vi "参数设置页.vi"() -> ()   [LabVIEW 2016, in "斯坦道CODMn.lvlib"]
panel:
  in  "手动模式":bool
  in  "采水泵排液时间/s:":i32
  in  "采水泵沉淀时间/s:":i32
  in  "采水泵润洗时间/s:":i32
  in  "采水泵进样时间/s:":i32
  in  "标度泵计量数 2":dbl
  in  "零点泵计量数 2":dbl
  in  "氢氧化钠:":dbl
  in  "屏蔽负值":bool
  in  "常规版/认证版":enum16{"常规版-酸性", "常规版-碱性", "认证版", "浮台版"}(ring)
  out "稀释倍数解释":string
  in  "CODMn零点核查选择":enum16{"零点核查走纯水管", "零点核查走零漂管"}(ring)
  in  "低量程稀释倍数:":dbl=1.0
  in  "高量程稀释倍数:":dbl=2.0
  in  "零点液自动补测":bool
  in  "跨度液自动补测":bool
  in  "标准液自动补测":bool
  in  "零点液偏差":dbl
  in  "跨度液偏差":dbl
  in  "标准液偏差":dbl
  in  "更换泵管":bool
  in  "跨度值":dbl
  in  "加标回收量程：":enum32{"H", "L", "AUTO"}(ring)=enum."AUTO"
  out "CODMn序列号":string
  out "CODMn软件版本：":string
  in  "标样核查量程选择":enum32{"H", "L", "AUTO"}(ring)=enum."AUTO"
  in  "标样浓度":dbl
  in  "零点核查量程选择":enum32{"H", "L", "AUTO"}(ring)=enum."AUTO"
  in  "零点核查浓度":dbl
  in  "跨度量程选择":enum32{"H", "L", "AUTO"}(ring)=enum."AUTO"
  in  "跨度液浓度":dbl
  in  "水样：":dbl
  in  "蒸馏水：":dbl
  in  "标液：":dbl
  in  "零点核查样：":dbl
  in  "加标回收样：":dbl
  in  "草酸钠":dbl
  in  "高锰酸钾":dbl
  in  "硫酸":dbl
  out "量程解释说明":string
  in  "高切低阈值:":dbl
  in  "低切高阈值:":dbl
  in  "水样量程选择:":enum16{"L", "H", "自动切换测一次", "自动切换测两次"}(ring)
  in  "标准液浓度":dbl
  in  "温度":dbl
  in  "恒温时间":dbl
  in  "当前量程：":enum16{"L", "H"}(ring)
  # "基本参数设置"
  # "泵计量参数设置"
  # "高锰酸钾："
  # "加热恒温温度(℃):"
  # "草酸钠："
  # "恒温时间(分钟):"
  # "硫酸："
  # "标准液浓度(mg/L):"
  # "跨度核查浓度："
  # "零点液偏差±:"
  # "标准液偏差%:"
  # "跨度核查量程："
  # "跨度液偏差%:"
  # "零点核查浓度："
  # "标样浓度："
  # "零点核查量程："
  # "标样核查量程："
  # "跨度值:"
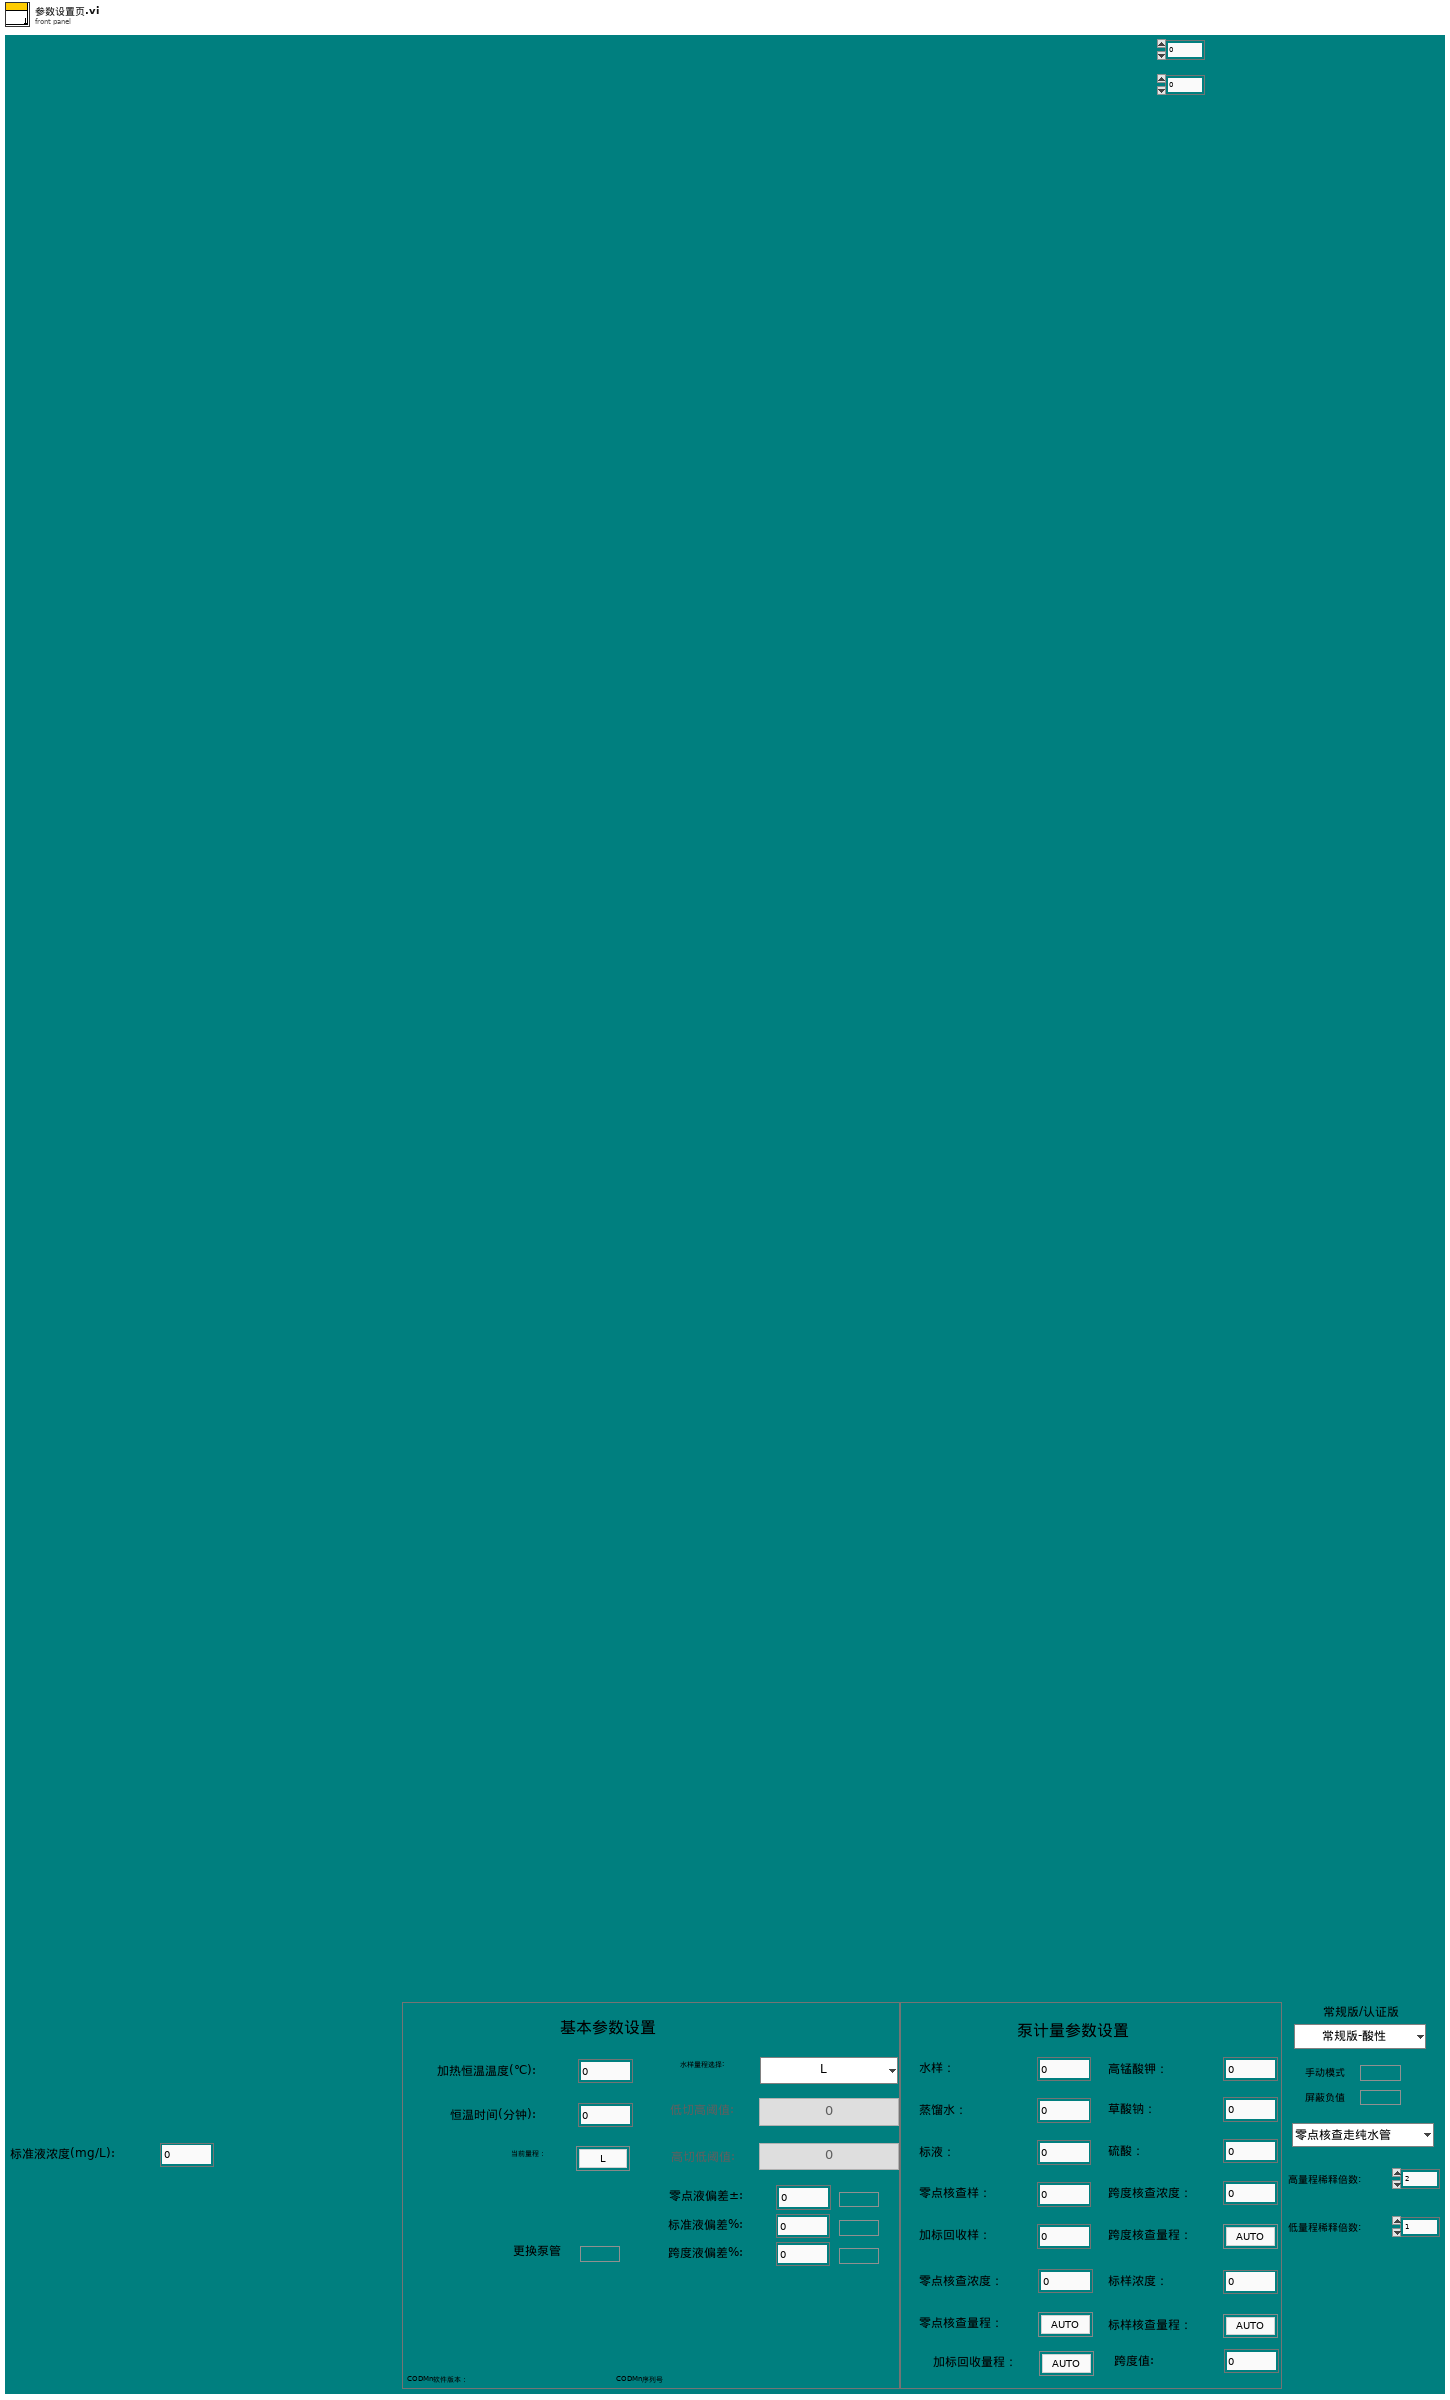
[diagram p1: front panel]
types:
  T1 = cluster{"时间":timestamp, "水样计量数":u16, "蒸馏水计量数":u16, "标液计量数":u16, "零点核查计量数":u16, "加标回收计量数":u16, "硫酸计量数":u16, "高锰酸钾计量数":u16, "草酸钠计量数":u16, "更换泵管":string}
  T2 = cluster{"测量量程":dbl, "测量精度":dbl, "测量间隔":dbl, "消解温度":dbl, "消解时长":dbl, "空白校准时间":timestamp, "曲线截距":dbl, "曲线斜率":dbl, "测量检出限":dbl, "测量信号值":dbl, "线性相关系数":dbl, "二次多项式系数":dbl, "标样校准时间":timestamp, "稀释倍数":dbl, "三项式系数":dbl, "空白标定系数":dbl, "量程系数":dbl, "F0/ORPA":dbl, "F1/ORPB":dbl, "F2/ORPK":dbl, "F3":dbl, "F4":dbl, "F5":dbl, "F6":dbl, "F7":dbl, "X0/滴定数":dbl, "量程":dbl}
  T3 = enum8{"Enabled", "Disabled", "Disabled and Grayed Out"}
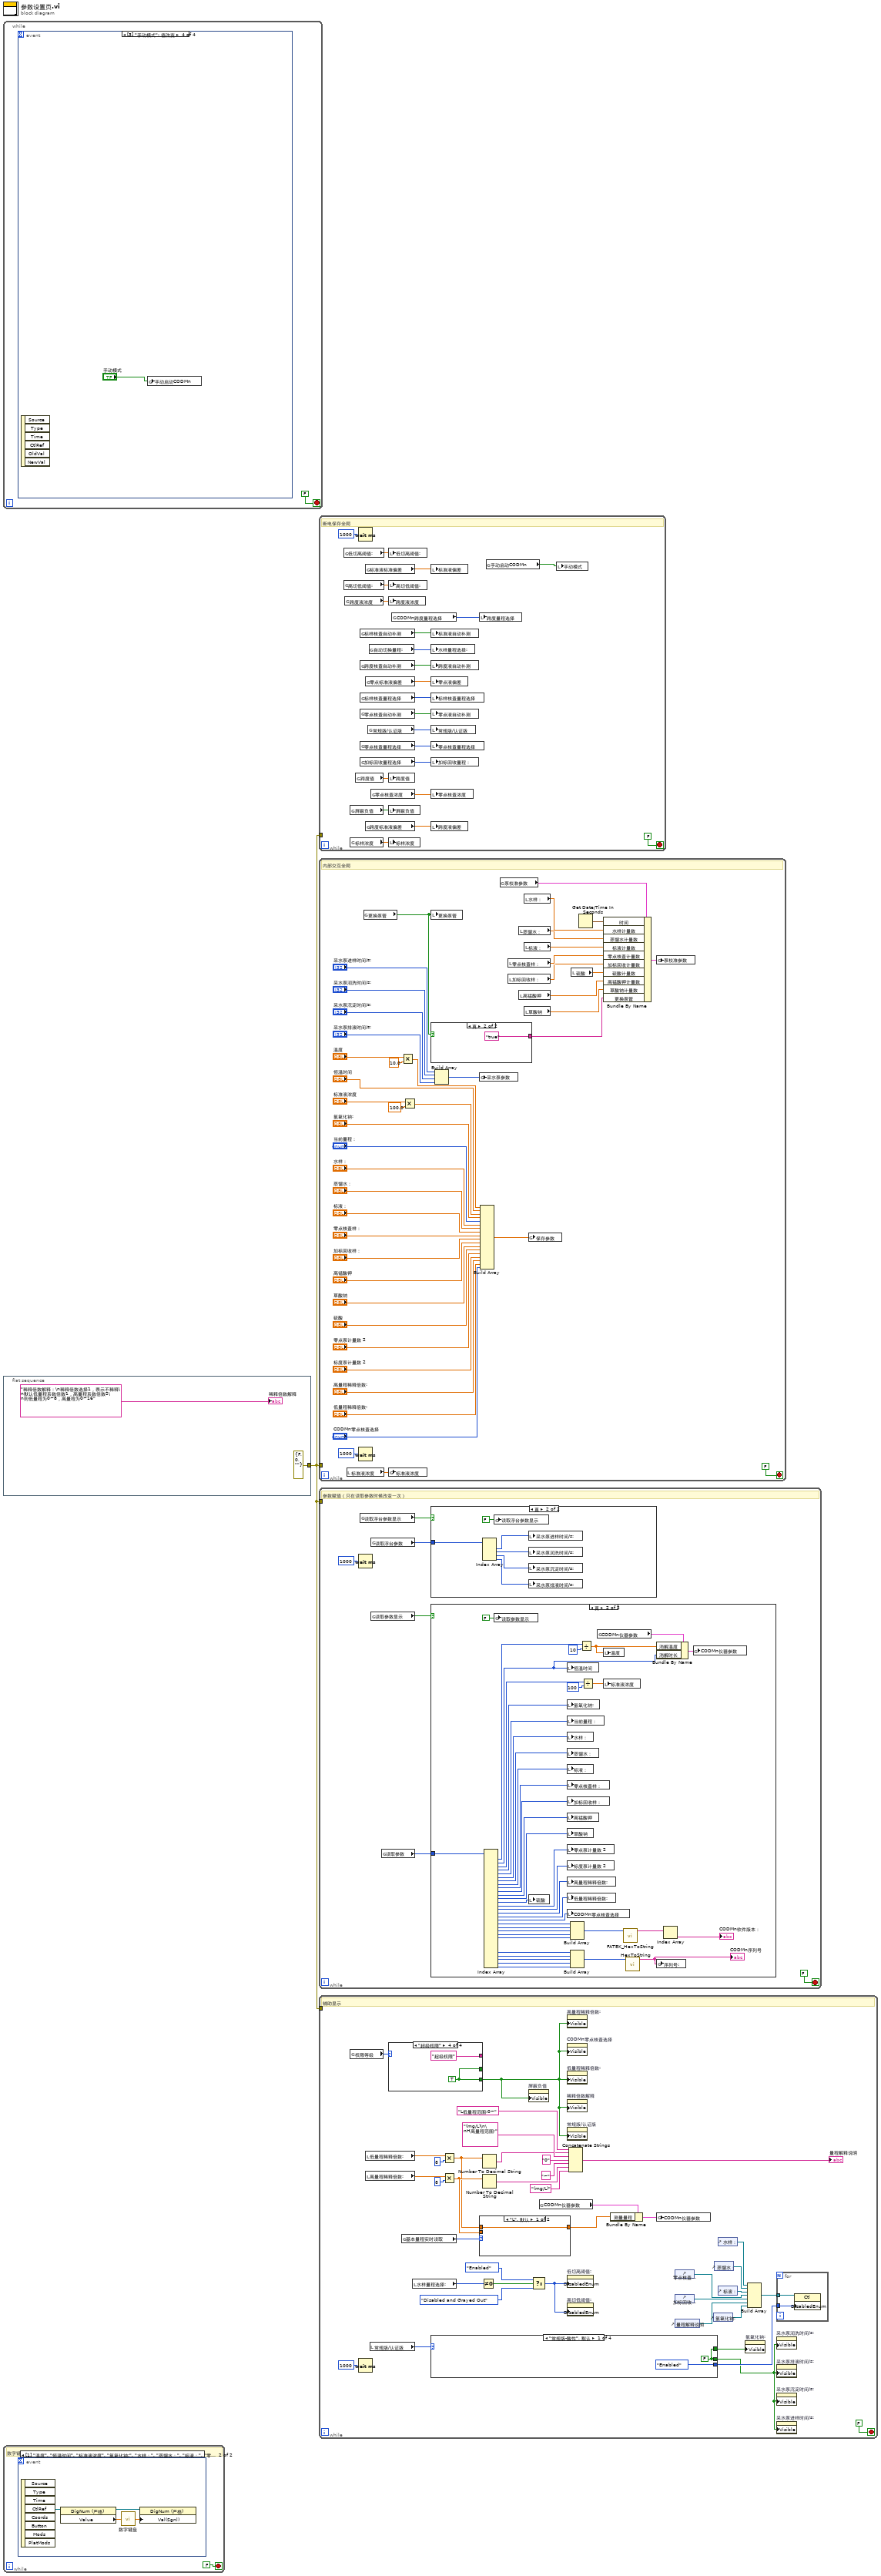
[diagram p0: block diagram]
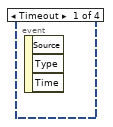
[diagram p2: hidden frame]
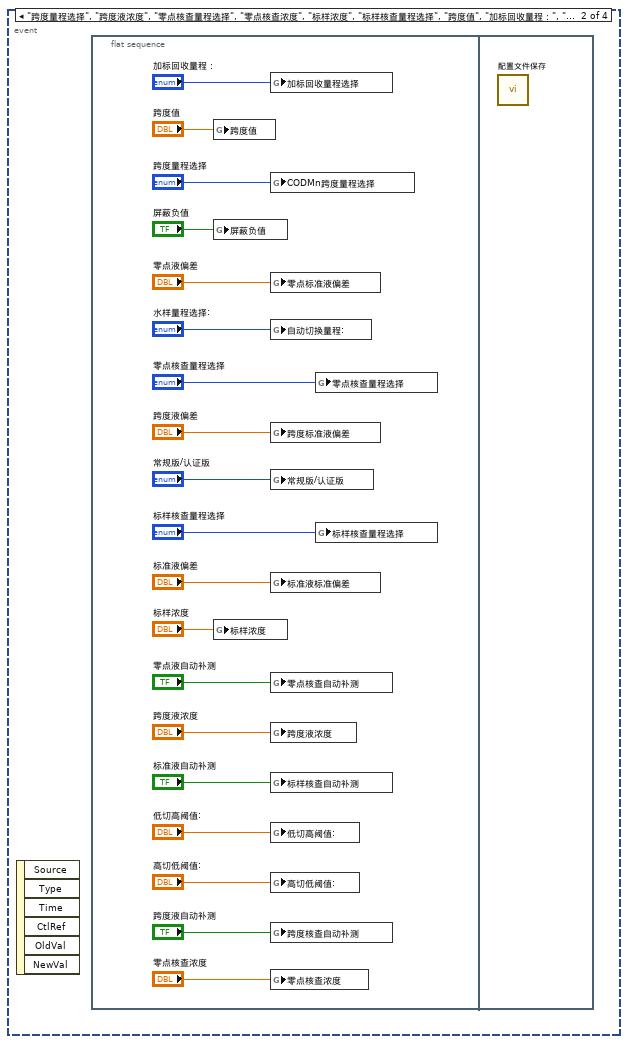
[diagram p3: hidden frame]
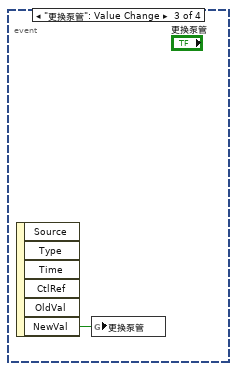
[diagram p4: hidden frame]
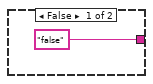
[diagram p7: hidden frame]
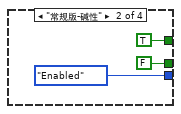
[diagram p8: hidden frame]
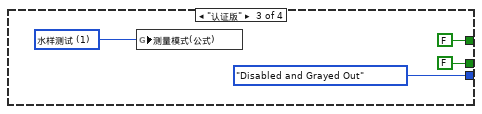
[diagram p9: hidden frame]
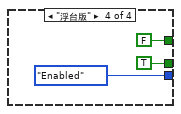
[diagram p10: hidden frame]
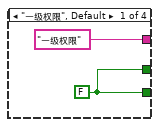
[diagram p11: hidden frame]
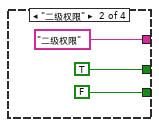
[diagram p12: hidden frame]
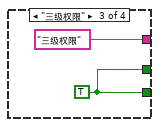
[diagram p13: hidden frame]
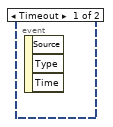
[diagram p15: hidden frame]
diagram:
  n1 = while {
    stop <- FALSE stop-if-true
    n2 = event shown="[3] \"手动模式\": 值改变" {
      selector: _ -> [_ _ _ _]
      dyn-events: _ -> [_ _ _ _]
      timeout: _ -> [_ _ _ _]
      event Timeout {
        n3 = event-data() -> ()  [unwired: 1 in, 3 out]
      }
      event "跨度量程选择", "跨度液浓度", "零点核查量程选择", "零点核查浓度", "标样浓度", "标样核查量程选择", "跨度值", "加标回收量程：", "标准液偏差", "跨度液偏差", "零点液偏差", "标准液自动补测", "跨度液自动补测", "零点液自动补测", "常规版/认证版", "屏蔽负值", "水样量程选择:", "低切高阈值:", "高切低阈值:": Value Change {
        n4 = event-data() -> ()  [unwired: 1 in, 6 out]
        n5 = flat-sequence {
          frame #0 {
            n6 = global write "CODMn断电保存全局变量.vi" "跨度值"("跨度值") -> ()
            n7 = global write "CODMn断电保存全局变量.vi" "屏蔽负值"("屏蔽负值") -> ()
            n8 = global write "CODMn断电保存全局变量.vi" "标样浓度"("标样浓度") -> ()
            n9 = global write "CODMn断电保存全局变量.vi" "加标回收量程选择"("加标回收量程：") -> ()
            n10 = global write "CODMn断电保存全局变量.vi" "CODMn跨度量程选择"("跨度量程选择") -> ()
            n11 = global write "CODMn断电保存全局变量.vi" "零点标准液偏差"("零点液偏差") -> ()
            n12 = global write "CODMn断电保存全局变量.vi" "自动切换量程:"("水样量程选择:") -> ()
            n13 = global write "CODMn断电保存全局变量.vi" "跨度标准液偏差"("跨度液偏差") -> ()
            n14 = global write "CODMn断电保存全局变量.vi" "常规版/认证版"("常规版/认证版") -> ()
            n15 = global write "CODMn断电保存全局变量.vi" "标准液标准偏差"("标准液偏差") -> ()
            n16 = global write "CODMn断电保存全局变量.vi" "零点核查自动补测"("零点液自动补测") -> ()
            n17 = global write "CODMn断电保存全局变量.vi" "跨度液浓度"("跨度液浓度") -> ()
            n18 = global write "CODMn断电保存全局变量.vi" "标样核查自动补测"("标准液自动补测") -> ()
            n19 = global write "CODMn断电保存全局变量.vi" "低切高阈值:"("低切高阈值:") -> ()
            n20 = global write "CODMn断电保存全局变量.vi" "高切低阈值:"("高切低阈值:") -> ()
            n21 = global write "CODMn断电保存全局变量.vi" "跨度核查自动补测"("跨度液自动补测") -> ()
            n22 = global write "CODMn断电保存全局变量.vi" "零点核查浓度"("零点核查浓度") -> ()
            n23 = global write "CODMn断电保存全局变量.vi" "零点核查量程选择"("零点核查量程选择") -> ()
            n24 = global write "CODMn断电保存全局变量.vi" "标样核查量程选择"("标样核查量程选择") -> ()
          }
          frame #1 {
            n25 = call "配置文件保存.vi"() -> ()  [unwired: 12 in]
          }
        }
      }
      event "更换泵管": Value Change {
        n26 = event-data() -> ("NewVal"=w22:bool)  [unwired: 1 in, 5 out]
        n27 = global write "COD内部交互全局.vi" "更换泵管"(w22) -> ()
      }
      event "手动模式": Value Change {
        n28 = event-data() -> ()  [unwired: 1 in, 6 out]
        n29 = global write "CODMN外部API.vi" "手动启动CODMn"("手动模式") -> ()
      }
    }
  }
  n30 = flat-sequence {
    tunnel: [errorcluster {"status"=FALSE, "code"=0, "source"=""} ("error out")] -> w1
    frame #0 {
      "稀释倍数解释" <- "稀释倍数解释：\n稀释倍数选择1，表示不稀释\n默认低量程系数倍数1，高量程系数倍数2\n则低量程为0~8，高量程为0~16" ("稀释倍数解释")
    }
  }
  n31 = while {
    stop <- FALSE stop-if-true
    # "数字键盘输入"
    n32 = event shown="[1] \"温度\", \"恒温时间\", \"标准液浓度\", \"氢氧化钠:\", \"水样：\", \"蒸馏水：\", \"标液：\", \"零点核查样：\", \"加标回收样：\", \"草酸钠\", \"高锰酸钾\", \"硫酸\", \"高量程稀释倍数:\", \"低量程稀释倍数:\", \"跨度液浓度\", \"零点核查浓度\", \"标样浓度\", \"标准液偏差\", \"跨度液偏差\", \"零点液偏差\", \"低切高阈值:\", \"高切低阈值:\": 鼠标按下" {
      selector: _ -> [_ _]
      dyn-events: _ -> [_ _]
      timeout: _ -> [_ _]
      event Timeout {
        n33 = event-data() -> ()  [unwired: 1 in, 3 out]
      }
      event "温度", "恒温时间", "标准液浓度", "氢氧化钠:", "水样：", "蒸馏水：", "标液：", "零点核查样：", "加标回收样：", "草酸钠", "高锰酸钾", "硫酸", "高量程稀释倍数:", "低量程稀释倍数:", "跨度液浓度", "零点核查浓度", "标样浓度", "标准液偏差", "跨度液偏差", "零点液偏差", "低切高阈值:", "高切低阈值:": Mouse Down {
        n34 = event-data() -> ("CtlRef"=w30:refnum<vi>)  [unwired: 1 in, 7 out]
        n35 = property class="DigNum (严格)"(reference=w30) -> (reference out=w28:refnum<vi>, "Value"=w29:dbl)  [unwired: 1 in, 1 out]
        n36 = call "数字键盘.vi"("OldNumber"=w29) -> ("NewNumber"=w27:sgl)
        n37 = property class="DigNum (严格)"(reference=w28, "Val(Sgnl)"=w27) -> ()  [unwired: 1 in, 2 out]
      }
    }
  }
  n38 = while {
    tunnel: w1 -> [_]
    stop <- FALSE stop-if-true
    # "断电保存全局"
    n39 = global read "CODMn断电保存全局变量.vi" "低切高阈值:"() -> (w50:dbl)
    n40 = global read "CODMn断电保存全局变量.vi" "高切低阈值:"() -> (w49:dbl)
    n41 = global read "CODMn断电保存全局变量.vi" "跨度液浓度"() -> (w33:dbl)
    n42 = global read "CODMn断电保存全局变量.vi" "屏蔽负值"() -> (w44:bool)
    n43 = global read "CODMn断电保存全局变量.vi" "标样浓度"() -> (w32:dbl)
    n44 = global read "CODMn断电保存全局变量.vi" "跨度值"() -> (w34:dbl)
    n45 = Wait (ms)(milliseconds to wait=u32 1000 ("等待时间（毫秒）")) -> ()  [unwired: 1 out]
    n46 = global read "CODMn断电保存全局变量.vi" "标样核查自动补测"() -> (w42:bool)
    n47 = global read "CODMn断电保存全局变量.vi" "跨度核查自动补测"() -> (w41:bool)
    n48 = global read "CODMn断电保存全局变量.vi" "标样核查量程选择"() -> (w47:enum32{"H", "L", "AUTO"})
    n49 = global read "CODMn断电保存全局变量.vi" "零点核查自动补测"() -> (w43:bool)
    n50 = global read "CODMn断电保存全局变量.vi" "零点核查量程选择"() -> (w37:enum32{"H", "L", "AUTO"})
    n51 = global read "CODMn断电保存全局变量.vi" "加标回收量程选择"() -> (w36:enum32{"H", "L", "AUTO"})
    n52 = global read "CODMn断电保存全局变量.vi" "标准液标准偏差"() -> (w40:dbl)
    n53 = global read "CODMn断电保存全局变量.vi" "零点标准液偏差"() -> (w39:dbl)
    n54 = global read "CODMn断电保存全局变量.vi" "跨度标准液偏差"() -> (w38:dbl)
    n55 = global read "CODMn断电保存全局变量.vi" "常规版/认证版"() -> (w45:enum16{"常规版-酸性", "常规版-碱性", "认证版", "浮台版"})
    n56 = global read "CODMn断电保存全局变量.vi" "自动切换量程:"() -> (w48:enum16{"L", "H", "自动切换测一次", "自动切换测两次"})
    n57 = global read "CODMn断电保存全局变量.vi" "零点核查浓度"() -> (w35:dbl)
    n58 = local write "低切高阈值:"(w50) -> ()
    n59 = local write "高切低阈值:"(w49) -> ()
    n60 = local write "跨度液浓度"(w33) -> ()
    n61 = local write "跨度值"(w34) -> ()
    n62 = local write "屏蔽负值"(w44) -> ()
    n63 = local write "标样浓度"(w32) -> ()
    n64 = global read "CODMn断电保存全局变量.vi" "CODMn跨度量程选择"() -> (w46:enum32{"H", "L", "AUTO"})
    n65 = local write "标准液偏差"(w40) -> ()
    n66 = local write "标准液自动补测"(w42) -> ()
    n67 = local write "水样量程选择:"(w48) -> ()
    n68 = local write "跨度液自动补测"(w41) -> ()
    n69 = local write "零点液偏差"(w39) -> ()
    n70 = local write "标样核查量程选择"(w47) -> ()
    n71 = local write "零点液自动补测"(w43) -> ()
    n72 = local write "常规版/认证版"(w45) -> ()
    n73 = local write "零点核查量程选择"(w37) -> ()
    n74 = local write "加标回收量程："(w36) -> ()
    n75 = local write "零点核查浓度"(w35) -> ()
    n76 = local write "跨度液偏差"(w38) -> ()
    n77 = local write "跨度量程选择"(w46) -> ()
    n78 = global read "CODMN外部API.vi" "手动启动CODMn"() -> (w31:bool)
    n79 = local write "手动模式"(w31) -> ()
  }
  n80 = while {
    tunnel: w1 -> [_]
    stop <- FALSE stop-if-true
    # "内部交互全局"
    n81 = local read "标准液浓度"() -> (w94:dbl)
    n82 = Wait (ms)(milliseconds to wait=u32 1000 ("等待时间（毫秒）")) -> ()  [unwired: 1 out]
    n83 = global read "COD内部交互全局.vi" "更换泵管"() -> (w53:bool)
    n84 = global write "COD浓度全局变量.vi" "标准液浓度"(w94) -> ()
    n85 = Multiply(x="温度", y=10.0) -> (x*y=w74:dbl)
    n86 = Multiply(x="标准液浓度", y=100.0) -> (x*y=w76:dbl)
    n87 = local write "更换泵管"(w53) -> ()
    n88 = case shown="真" w53 {
      tunnel: ["false" "true"] -> w62
      frame False {
      }
      frame True {
      }
    }
    n89 = Build Array("采水泵进样时间/s:", "采水泵润洗时间/s:", "采水泵沉淀时间/s:", "采水泵排液时间/s:") -> (w70:i32[])
    n90 = global write "COD内部交互全局.vi" "采水泵参数"(w70) -> ()
    n91 = Build Array(w74, "恒温时间", w76, "氢氧化钠:", "当前量程：", "水样：", "蒸馏水：", "标液：", "零点核查样：", "加标回收样：", "高锰酸钾", "草酸钠", "硫酸", "零点泵计量数 2", "标度泵计量数 2", "高量程稀释倍数:", "低量程稀释倍数:", "CODMn零点核查选择") -> (w77:dbl[])
    n92 = global read "COD内部交互全局.vi" "泵校准参数"() -> (w65:T1)
    n93 = local read "零点核查样："() -> (w58:dbl)
    n94 = local read "加标回收样："() -> (w57:dbl)
    n95 = local read "蒸馏水："() -> (w60:dbl)
    n96 = local read "高锰酸钾"() -> (w55:dbl)
    n97 = local read "水样："() -> (w61:dbl)
    n98 = local read "标液："() -> (w59:dbl)
    n99 = local read "草酸钠"() -> (w54:dbl)
    n100 = global write "COD内部交互全局.vi" "保存参数"(w77) -> ()
    n101 = local read "硫酸"() -> (w56:dbl)
    n102 = Get Date/Time In Seconds() -> (seconds since 1Jan1904=w63:timestamp)
    n103 = Bundle By Name(cluster=w65, "时间"=w63, "水样计量数"=w61, "蒸馏水计量数"=w60, "标液计量数"=w59, "零点核查计量数"=w58, "加标回收计量数"=w57, "硫酸计量数"=w56, "高锰酸钾计量数"=w55, "草酸钠计量数"=w54, "更换泵管"=w62) -> (w64:T1)
    n104 = global write "COD内部交互全局.vi" "泵校准参数"(w64) -> ()
  }
  n105 = while {
    tunnel: w1 -> [_]
    stop <- FALSE stop-if-true
    # "参数赋值（只在读取参数时候改变一次）"
    n106 = Wait (ms)(milliseconds to wait=u32 1000 ("等待时间（毫秒）")) -> ()  [unwired: 1 out]
    n107 = global read "COD内部交互全局.vi" "读取浮台参数显示"() -> (w103:bool)
    n108 = global read "COD内部交互全局.vi" "读取浮台参数"() -> (w102:u16[])
    n109 = global read "COD内部交互全局.vi" "读取参数显示"() -> (w100:bool)
    n110 = global read "COD内部交互全局.vi" "读取参数"() -> (w99:u16[])
    n111 = case shown="真" w103 {
      tunnel: w102 -> [_ w150]
      frame False {
      }
      frame True {
        n112 = Index Array(array=w150) -> (element #1=w149:u16, element #2=w148:u16, element #3=w147:u16, element #4=w146:u16)  [unwired: 4 in]
        n113 = global write "COD内部交互全局.vi" "读取浮台参数显示"(FALSE ("读取参数显示")) -> ()
        n114 = local write "采水泵进样时间/s:"(w149) -> ()
        n115 = local write "采水泵润洗时间/s:"(w148) -> ()
        n116 = local write "采水泵沉淀时间/s:"(w147) -> ()
        n117 = local write "采水泵排液时间/s:"(w146) -> ()
      }
    }
    n118 = case shown="真" w100 {
      tunnel: w99 -> [_ w144]
      frame False {
      }
      frame True {
        n119 = Index Array(array=w144) -> (element #1=w142:u16, element #2=w138:u16, element #3=w136:u16, element #4=w134:u16, element #5=w133:u16, element #6=w132:u16, element #7=w131:u16, element #8=w130:u16, element #9=w129:u16, element #10=w128:u16, element #11=w127:u16, element #12=w126:u16, element #13=w125:u16, element #14=w124:u16, element #15=w123:u16, element #16=w122:u16, element #17=w121:u16, element #18=w115:u16, element #19=w114:u16, element #20=w113:u16, element #21=w112:u16, element #22=w111:u16, element #23=w110:u16, element #27=w109:u16, element #28=w108:u16, element #29=w107:u16, element #30=w106:u16, element #31=w105:u16)  [unwired: 31 in, 3 out]
        n120 = global write "COD内部交互全局.vi" "读取参数显示"(FALSE ("读取参数显示")) -> ()
        n121 = local write "硫酸"(w125) -> ()
        n122 = local write "恒温时间"(w138) -> ()
        n123 = local write "氢氧化钠:"(w134) -> ()
        n124 = local write "当前量程："(w133) -> ()
        n125 = local write "水样："(w132) -> ()
        n126 = local write "蒸馏水："(w131) -> ()
        n127 = local write "标液："(w130) -> ()
        n128 = local write "零点核查样："(w129) -> ()
        n129 = local write "加标回收样："(w128) -> ()
        n130 = local write "高锰酸钾"(w127) -> ()
        n131 = local write "草酸钠"(w126) -> ()
        n132 = local write "零点泵计量数 2"(w124) -> ()
        n133 = local write "标度泵计量数 2"(w123) -> ()
        n134 = local write "高量程稀释倍数:"(w122) -> ()
        n135 = local write "低量程稀释倍数:"(w121) -> ()
        n136 = local write "CODMn零点核查选择"(w115) -> ()
        n137 = Build Array(w114, w113, w112, w111, w110) -> (w120:u16[])
        n138 = Build Array(w109, w108, w107, w106, w105) -> (w119:u16[])
        n139 = Divide(x=w142, y=u16 10) -> (x/y=w139:dbl)
        n140 = Divide(x=w136, y=u16 100) -> (x/y=w135:dbl)
        n141 = global read "CODMn断电保存全局变量.vi" "CODMn仪器参数"() -> (w141:T2)
        n142 = local write "温度"(w139) -> ()
        n143 = local write "标准液浓度"(w135) -> ()
        n144 = call "FATEK_HexToString.vi"("数组"=w120) -> ("STRING"=w118:string[])  [unwired: 10 in]
        n145 = call "HexToString.vi"("数组"=w119) -> ("字符串"=w116:string)  [unwired: 10 in]
        "CODMn序列号" <- w116
        n146 = Bundle By Name(cluster=w141, "消解温度"=w139, "消解时长"=w138) -> (w140:T2)
        n147 = global write "COD内部交互全局.vi" "序列号:"(w116) -> ()
        n148 = Index Array(array=w118) -> (element=→"CODMn软件版本：":string)  [unwired: 1 in]
        n149 = global write "CODMn断电保存全局变量.vi" "CODMn仪器参数"(w140) -> ()
      }
    }
  }
  n150 = while {
    tunnel: w1 -> [_]
    stop <- FALSE stop-if-true
    # "辅助显示"
    n151 = global read "CODMN外部API.vi" "权限等级"() -> (w170:enum16{"一级权限", "二级权限", "三级权限", "超级权限"})
    n152 = Wait (ms)(milliseconds to wait=u32 1000 ("等待时间（毫秒）")) -> ()  [unwired: 1 out]
    n153 = local read "低量程稀释倍数:"() -> (w186:dbl)
    n154 = local read "高量程稀释倍数:"() -> (w178:dbl)
    n155 = local read "常规版/认证版"() -> (w160:enum16{"常规版-酸性", "常规版-碱性", "认证版", "浮台版"})
    n156 = case shown="\"超级权限\"" w170 {
      tunnel: [w205 FALSE w210 w212] -> w169
      tunnel: ["一级权限" "二级权限" "三级权限" "超级权限"] -> _
      tunnel: [w205 TRUE w210 w212] -> _
      frame "一级权限", Default {
        w205 = FALSE
      }
      frame "二级权限" {
      }
      frame "三级权限" {
        w210 = TRUE
      }
      frame "超级权限" {
        w212 = TRUE
      }
    }
    n157 = global read "COD内部交互全局.vi" "基本量程实时读取"() -> (w174:enum16{"L", "H", "AUTO"})
    n158 = local read "水样量程选择:"() -> (w153:enum16{"L", "H", "自动切换测一次", "自动切换测两次"})
    n159 = case shown="\"常规版-酸性\", 默认" w160 {
      tunnel: [T3."Enabled" ("禁用") T3."Enabled" ("禁用") T3."Disabled and Grayed Out" ("禁用") T3."Enabled" ("禁用")] -> w159
      tunnel: [w191 TRUE FALSE FALSE] -> w158
      tunnel: [w191 FALSE FALSE TRUE] -> w157
      frame "常规版-酸性", Default {
        w191 = FALSE
      }
      frame "常规版-碱性" {
      }
      frame "认证版" {
        w198 = u16 1 items=["水样测试"=1, "标样核查"=2, "零点核查"=3, "跨度核查"=4, "空白测试"=5, "平行样"=6, "加标回收"=7] ("测量模式(公式)")
        n160 = global write "CODMn断电保存全局变量.vi" "测量模式(公式)"(w198) -> ()
      }
      frame "浮台版" {
      }
    }
    n161 = Multiply(x=w186, y=i8 8) -> (x*y=w172:dbl)
    n162 = Multiply(x=w178, y=i8 8) -> (x*y=w173:dbl)
    n163 = case shown="\"L\", 默认" w174 {
      tunnel: w173 -> [_ w215]
      tunnel: [w214 w215] -> w171
      tunnel: w172 -> [w214 _]
      frame "L", Default {
      }
      frame "H" {
      }
    }
    n164 = Not Equal To 0?(x=w153) -> (x != 0?=w154:bool)
    n165 = Number To Decimal String(number=w172) -> (decimal integer string=w183:string)  [unwired: 1 in]
    n166 = Number To Decimal String(number=w173) -> (decimal integer string=w181:string)  [unwired: 1 in]
    n167 = property on="屏蔽负值" class="Bool (严格)"("Visible"=w169) -> ()  [unwired: 2 in, 2 out]
    n168 = Select(t=T3."Enabled" ("禁用"), s=w154, f=T3."Disabled and Grayed Out" ("禁用")) -> (s? t:f=w152:T3)
    n169 = global read "CODMn断电保存全局变量.vi" "CODMn仪器参数"() -> (w176:T2)
    n170 = property on="高量程稀释倍数:" class="DigNum (严格)"("Visible"=w169) -> ()  [unwired: 2 in, 2 out]
    n171 = property on="CODMn零点核查选择" class="Enum (严格)"("Visible"=w169) -> ()  [unwired: 2 in, 2 out]
    n172 = property on="低量程稀释倍数:" class="DigNum (严格)"("Visible"=w169) -> ()  [unwired: 2 in, 2 out]
    n173 = property on="稀释倍数解释" class="Str"("Visible"=w169) -> ()  [unwired: 2 in, 2 out]
    n174 = property on="常规版/认证版" class="Enum (严格)"("Visible"=w169) -> ()  [unwired: 2 in, 2 out]
    n175 = property on="低切高阈值:" class="DigNum (严格)"("DisabledEnum"=w152) -> ()  [unwired: 2 in, 2 out]
    n176 = property on="高切低阈值:" class="DigNum (严格)"("DisabledEnum"=w152) -> ()  [unwired: 2 in, 2 out]
    n177 = Concatenate Strings("L低量程范围:0~" ("量程解释说明"), w183, "(mg/L)\n\nH高量程范围:" ("量程解释说明"), "0" ("字符串"), "~" ("量程解释说明"), w181, "(mg/L)" ("量程解释说明")) -> (→"量程解释说明":string)
    n178 = Bundle By Name(cluster=w176, "测量量程"=w171) -> (w175:T2)
    n179 = global write "CODMn断电保存全局变量.vi" "CODMn仪器参数"(w175) -> ()
    n180 = control-ref of="零点核查样："() -> (w165:refnum<vi>)
    n181 = control-ref of="加标回收样："() -> (w164:refnum<vi>)
    n182 = control-ref of="量程解释说明"() -> (w163:refnum<vi>)
    n183 = control-ref of="氢氧化钠:"() -> (w162:refnum<vi>)
    n184 = control-ref of="蒸馏水："() -> (w167:refnum<vi>)
    n185 = control-ref of="水样："() -> (w168:refnum<vi>)
    n186 = control-ref of="标液："() -> (w166:refnum<vi>)
    n187 = property on="氢氧化钠:" class="DigNum (严格)"("Visible"=w158) -> ()  [unwired: 2 in, 2 out]
    n188 = Build Array(w168, w167, w166, w165, w164, w163, w162) -> (w161:refnum<vi>[])
    n189 = for {
      tunnel: w161 -> [w204] mode=indexing
      tunnel: w159 -> [w203]
      n190 = property class="Ctl"(reference=w204, "DisabledEnum"=w203) -> ()  [unwired: 1 in, 2 out]
    }
    n191 = property on="采水泵润洗时间/s:" class="DigNum (严格)"("Visible"=w157) -> ()  [unwired: 2 in, 2 out]
    n192 = property on="采水泵排液时间/s:" class="DigNum (严格)"("Visible"=w157) -> ()  [unwired: 2 in, 2 out]
    n193 = property on="采水泵沉淀时间/s:" class="DigNum (严格)"("Visible"=w157) -> ()  [unwired: 2 in, 2 out]
    n194 = property on="采水泵进样时间/s:" class="DigNum (严格)"("Visible"=w157) -> ()  [unwired: 2 in, 2 out]
  }
